vi "Keithley Sample Number for IT.vi"(11 "Start":dbl=1.0) -> (2 "Array":dbl[](array[numeric]) format="%#.1f")   [LabVIEW 2017]
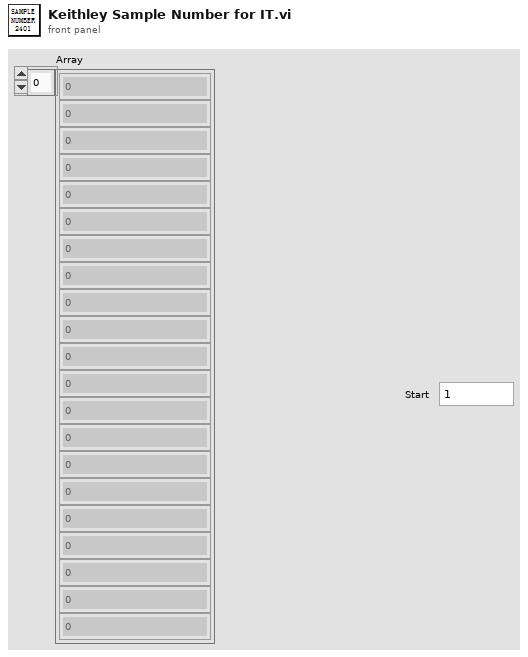
[diagram p1: front panel]
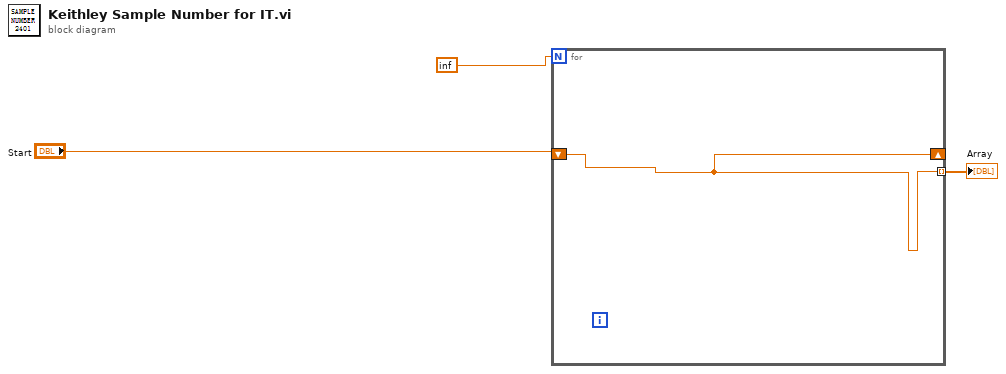
[diagram p0: block diagram]
diagram:
  n1 = for {
    N: inf -> [_]
    shift-right: [w4] -> _
    shift-left: "Start" -> [w4]
    tunnel: [w4] -> w2 mode=indexing
  }
  "Array" <- w2
